vi "Beam Profiler.vi"(7 "Image Ref":T2) -> ()   [LabVIEW 2016]
uses:
  <vilib>/vision/Image Controls.llb/IMAQ Image.ctl
  2D Gaussian Fit/2D Gaussian - Type Defs/2D Gaussian - Best Fit Parameters.ctl
  <vilib>/Utility/miscctls.llb/LVPointTypeDef.ctl
  <vilib>/vision/NI_Vision_Development_Module.lvlib
panel:
  out "Y FWHM (px)":dbl
  out "X FWHM (px)":dbl
  in  "Pixel Size (µm)":dbl=1.0
  out "Y FWHM (mm)":dbl
  out "X FWHM (mm)":dbl
  in  "Fitting On":bool
  out "Fit":dbl[][](graph)
  out "Best Fit Params":T1
  out "Image":u16[][](graph)
  in  "Update Rate (ms)":i32=50
  in  "Binning (pixels)":i32=10 min=1 step=1
  in  "Done":bool
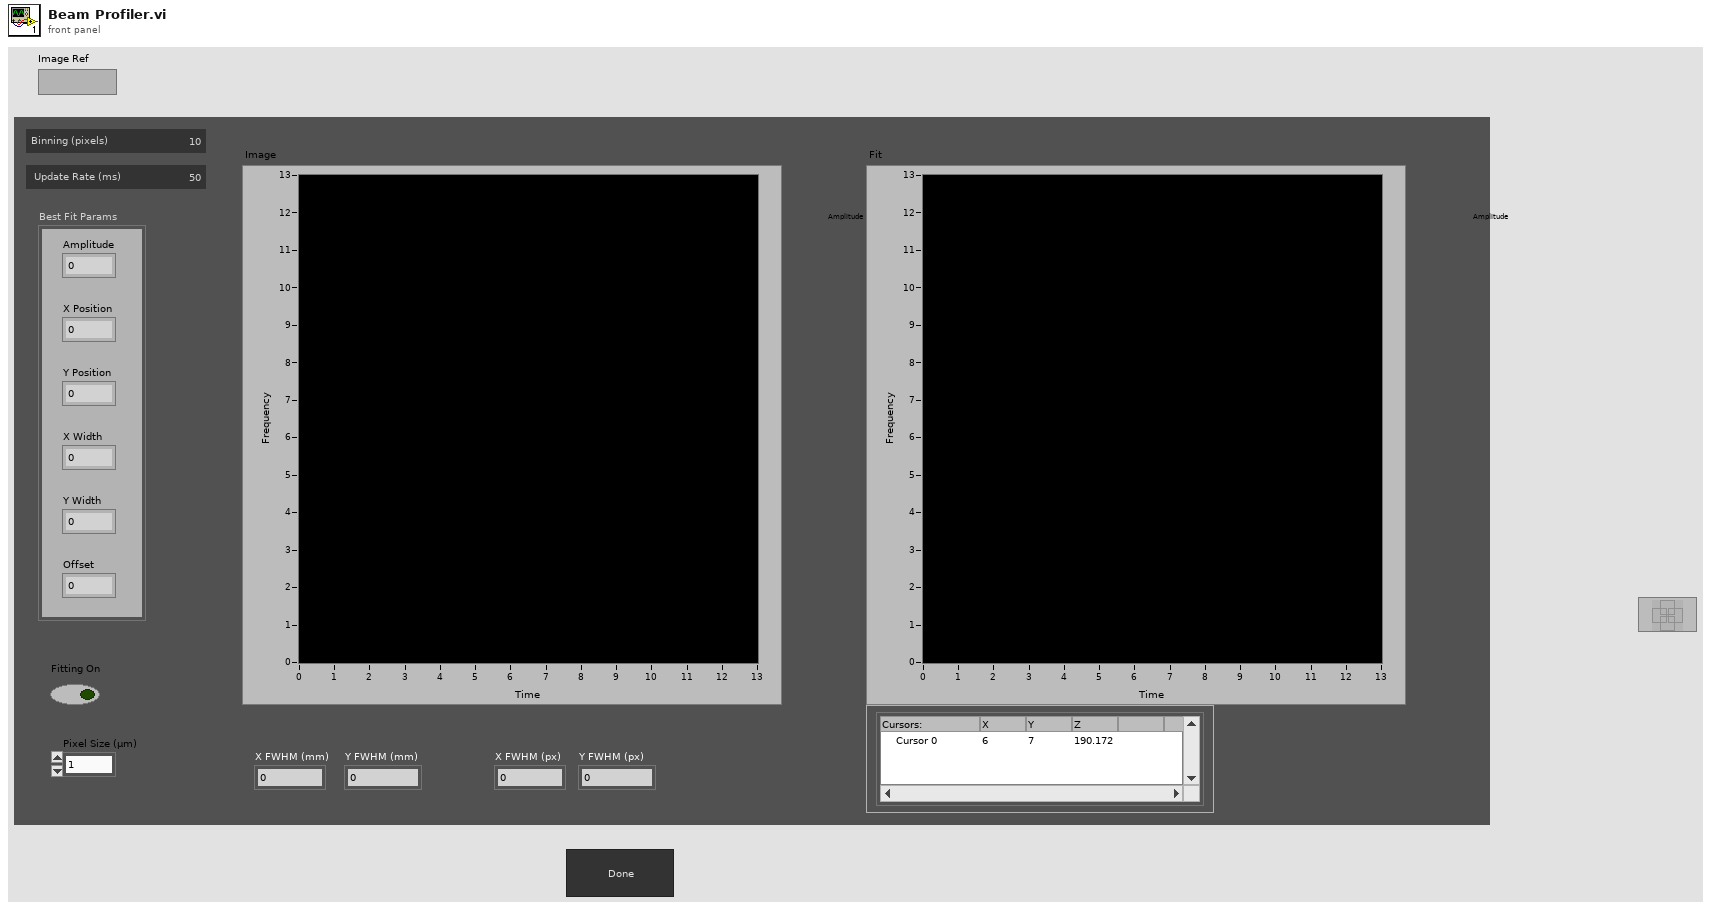
[diagram p1: front panel]
types:
  T1 = typedef "2D Gaussian - Best Fit Parameters.ctl" = cluster{"Amplitude":dbl, "X Position":dbl, "Y Position":dbl, "X Width":dbl, "Y Width":dbl, "Offset":dbl}
  T2 = typedef "IMAQ Image.ctl" = refnum<image>
  T3 = typedef "Image Type" = u32
  T4 = enum16{"Always On", "Always Off", "Off While Running"}
  T5 = typedef "LVPointTypeDef.ctl" = cluster{"Horizontal":i16, "Vertical":i16}
  T6 = typedef "LVRectTypeDef.ctl" = cluster{"Left":i16, "Top":i16, "Right":i16, "Bottom":i16}
  T7 = typedef "LVBoundsTypeDef.ctl" = cluster{"Width":u32, "Height":u32}
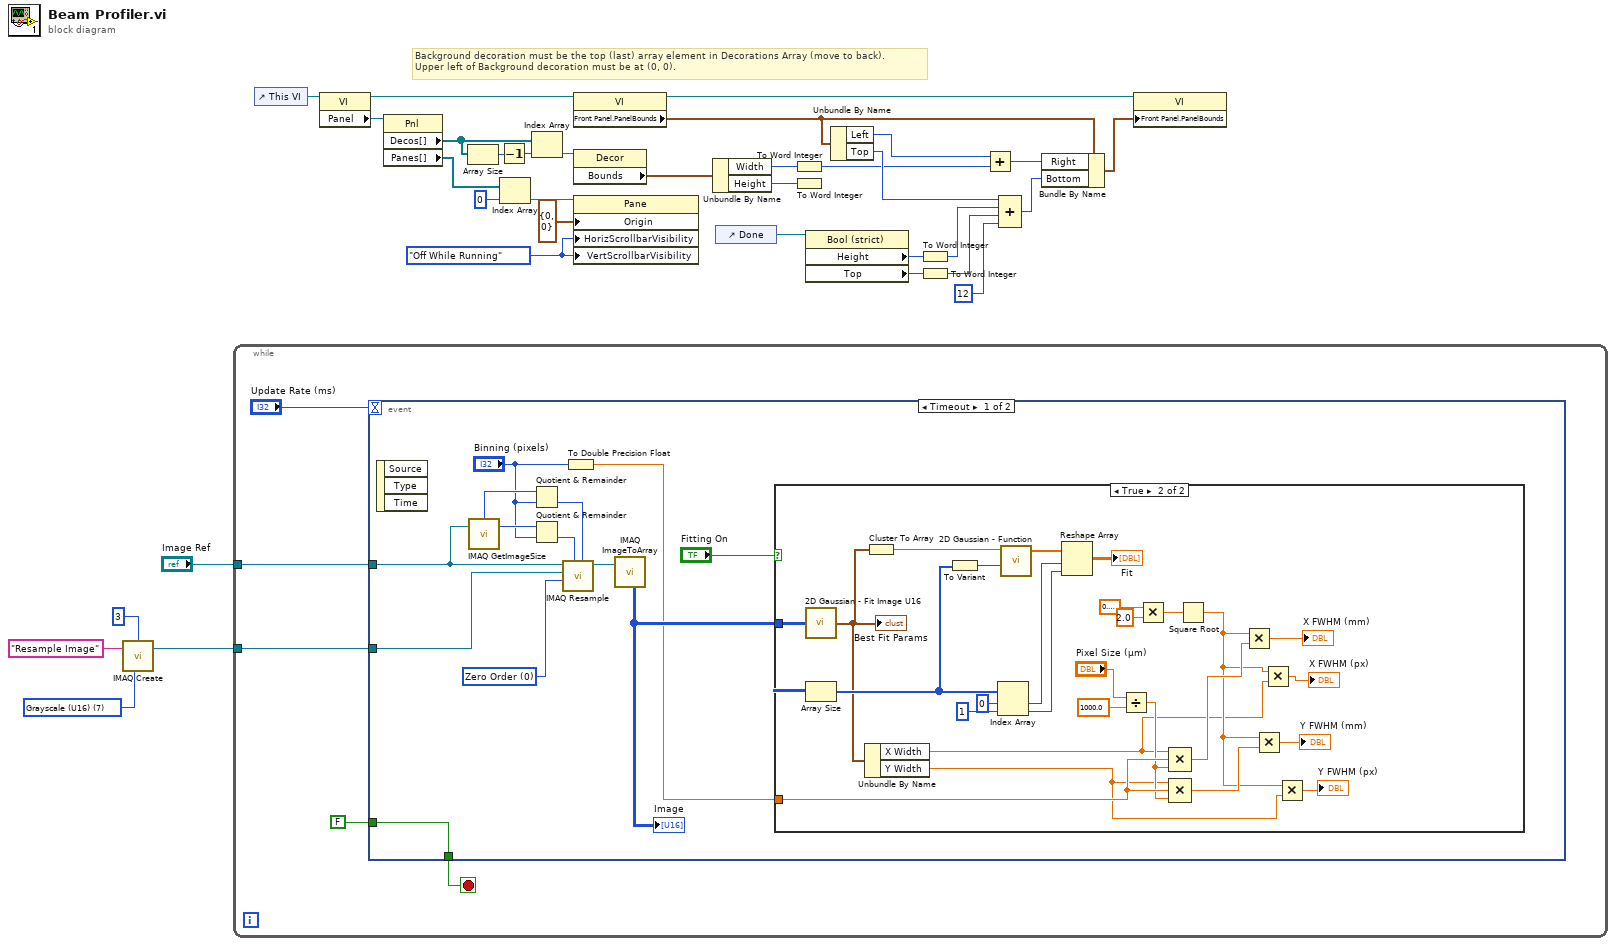
[diagram p0: block diagram]
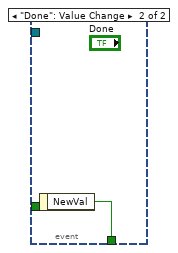
[diagram p3: hidden frame]
diagram:
  w4 = T3 7 items=["Grayscale (U8)", "Grayscale (I16)", "Grayscale (SGL)", "Complex (CSG)", "RGB (U32)", "HSL (U32)", "RGB (U64)", "Grayscale (U16)"] ("Image Type")
  w17 = T4."Off While Running" ("Vertical Scrollbar Visibility")
  # "Background decoration must be the top (last) array element in Decorations Array (move to back).\nUpper left of Background decoration must be at (0, 0)."
  n1 = call "IMAQ Create"("Border Size"=3, "Image Name"="Resample Image", "Image Type"=w4) -> ("New Image"=w1:T2)  [unwired: 2 in, 1 out]
  n2 = while {
    tunnel: "Image Ref" -> [w36]
    tunnel: w1 -> [w35]
    stop <- w38 stop-if-true
    n3 = event shown="[0] Timeout" {
      selector: _ -> [_ _]
      dyn-events: _ -> [_ _]
      timeout: "Update Rate (ms)" -> [_ _]
      tunnel: [w52 w80] -> w38
      tunnel: FALSE -> [w52 _]
      tunnel: w36 -> [w48 _]
      tunnel: w35 -> [w51 _]
      event Timeout {
        w50 = u32 0 items=["Zero Order", "Bi-Linear", "Quadratic", "Cubic Spline"] ("Interpolation Type")
        n4 = event-data() -> ()  [unwired: 1 in, 3 out]
        n5 = call "IMAQ GetImageSize"("Image"=w48) -> ("Y Resolution"=w46:i32, "X Resolution"=w47:i32)  [unwired: 3 in, 1 out]
        n6 = Quotient & Remainder(x=w47, y="Binning (pixels)") -> (floor(x/y)=w45:i32)  [unwired: 1 out]
        n7 = Quotient & Remainder(x=w46, y="Binning (pixels)") -> (floor(x/y)=w44:i32)  [unwired: 1 out]
        n8 = call "IMAQ Resample"("X Resolution"=w45, "Y Resolution"=w44, "Interpolation Type"=w50, "Image Dst"=w51, "Image Src"=w48) -> ("Image Dst Out"=w49:T2)  [unwired: 5 in, 1 out]
        n9 = To Double Precision Float(number="Binning (pixels)") -> (double precision float=w40:dbl)
        n10 = call "IMAQ ImageToArray"("Image"=w49) -> ("Image Pixels (U16)"=w43:u16[][])  [unwired: 3 in, 4 out]
        "Image" <- w43
        n11 = case shown="True" "Fitting On" {
          tunnel: w43 -> [_ w76]
          tunnel: w40 -> [_ w68]
          frame False {
          }
          frame True {
            n12 = call "2D Gaussian - Fit Image U16.vi"("Image In (U16)"=w76) -> ("Best Fit Params"=w69:T1)  [unwired: 13 in, 1 out]
            "Best Fit Params" <- w69
            n13 = Array Size(array=w76) -> (size(s)=w70:i32[])
            n14 = Unbundle By Name(w69) -> ("X Width"=w54:dbl, "Y Width"=w53:dbl)
            n15 = Cluster To Array(cluster=w69) -> (array=w79:dbl[])
            n16 = To Variant(anything=w70) -> (Variant=w71:variant)
            n17 = Index Array(array=w70, index #1=0 ("index"), index #2=1 ("index")) -> (element #1=w73:i32, element #2=w72:i32)
            n18 = call "2D Gaussian - Function.vi"("data"=w71, "a"=w79) -> ("f(X,a)"=w78:dbl[])  [unwired: 2 in, 2 out]
            n19 = Reshape Array(w78, w73, w72) -> (→"Fit":dbl[][])
            n20 = Divide(x="Pixel Size (µm)", y=1000.0) -> (x/y=w65:dbl)
            n21 = Multiply(x=0.6931471805599453, y=2.0) -> (x*y=w62:dbl)
            n22 = Compound Arithmetic op=MULTIPLY(w54, w68, w65) -> (w60:dbl)
            n23 = Compound Arithmetic op=MULTIPLY(w53, w68, w65) -> (w61:dbl)
            n24 = Square Root(x=w62) -> (sqrt(x)=w55:dbl)
            n25 = Multiply(x=w55, y=w60) -> (x*y=→"X FWHM (mm)":dbl)
            n26 = Multiply(x=w55, y=w61) -> (x*y=→"Y FWHM (mm)":dbl)
            n27 = Multiply(x=w55, y=w54) -> (x*y=→"X FWHM (px)":dbl)
            n28 = Multiply(x=w55, y=w53) -> (x*y=→"Y FWHM (px)":dbl)
          }
        }
      }
      event "Done": Value Change {
        n29 = event-data() -> ("NewVal"=w80:bool)  [unwired: 1 in]
      }
    }
  }
  n30 = control-ref of="This VI"() -> (w9:refnum<vi>)
  n31 = property class="VI"(reference=w9) -> (reference out=w18:refnum<vi>, "Panel"=w10:refnum<vi>)  [unwired: 1 in, 1 out]
  n32 = property class="Pnl"(reference=w10) -> ("Decos[]"=w8:refnum<vi>[], "Panes[]"=w14:refnum<vi>[])  [unwired: 1 in, 2 out]
  n33 = Array Size(array=w8) -> (size(s)=w6:i32)
  n34 = Decrement(x=w6) -> (x-1=w7:i32)
  n35 = Index Array(array=w14, index=0) -> (element=w13:refnum<vi>)
  n36 = Index Array(array=w8, index=w7) -> (element=w16:refnum<vi>)
  n37 = property class="VI"(reference=w18) -> (reference out=w20:refnum<vi>, "Front Panel.PanelBounds"=w21:T6)  [unwired: 1 in, 1 out]
  n38 = property class="Decor"(reference=w16) -> ("Bounds"=w19:T7)  [unwired: 1 in, 2 out]
  n39 = property class="Pane"(reference=w13, "Origin"=T5 {"Horizontal"=0, "Vertical"=0}, "HorizScrollbarVisibility"=w17, "VertScrollbarVisibility"=w17) -> ()  [unwired: 1 in, 2 out]
  n40 = Unbundle By Name(w19) -> ("Width"=w24:u32, "Height"=w27:u32)
  n41 = control-ref of="Done"() -> (w11:refnum<vi>)
  n42 = To Word Integer(number=w24) -> (16bit integer=w26:i16)
  n43 = To Word Integer(number=w27) -> ()  [unwired: 1 out]
  n44 = property class="Bool (strict)"(reference=w11) -> ("Height"=w29:u32, "Top"=w30:i32)  [unwired: 1 in, 2 out]
  n45 = Unbundle By Name(w21) -> ("Left"=w23:i16, "Top"=w34:i16)
  n46 = To Word Integer(number=w29) -> (16bit integer=w32:i16)
  n47 = To Word Integer(number=w30) -> (16bit integer=w33:i16)
  n48 = Add(x=w23, y=w26) -> (x+y=w25:i16)
  n49 = Compound Arithmetic op=ADD(w34, w32, w33, i16 12 ("y")) -> (w28:i16)
  n50 = Bundle By Name(cluster=w21, "Right"=w25, "Bottom"=w28) -> (w22:T6)
  n51 = property class="VI"(reference=w20, "Front Panel.PanelBounds"=w22) -> ()  [unwired: 1 in, 2 out]
